vi "Boolean_Create.vi"(7 "Object Attributes":T1, 8 "error in (no error)":errorcluster, 9 "BooleanControl Attributes":T3, 10 "Control Attributes":T4, 11 "Boolean In":refnum<class "Boolean.lvclass">) -> (0 "error out":errorcluster, 3 "Boolean Out":refnum<class "Boolean.lvclass">)   [LabVIEW 2015, in "Front Panel Publisher.lvlib" / "Boolean.lvclass"]
uses:
  Boolean.lvclass
  Control_class/Attributes.ctl
  Text_class/Text.lvclass
  Attributes.ctl
  Object_class/Attributes.ctl
  Object_class/Coordinates.ctl
  Control_class/Control.lvclass
  Object_class/Object.lvclass
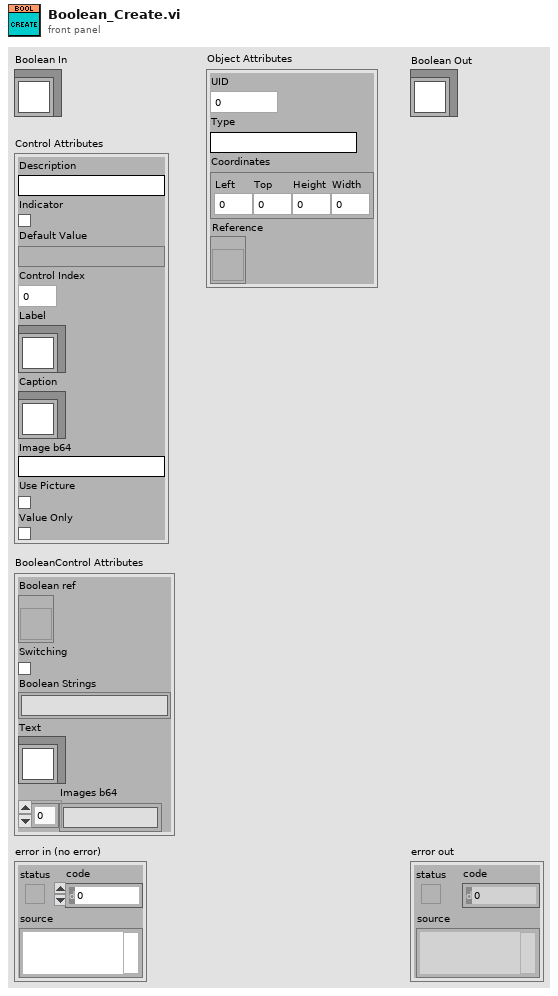
[diagram p1: front panel]
types:
  T1 = typedef "Front Panel Publisher.lvlib/Object.lvclass/Attributes.ctl" = cluster{"UID":i32, "Type":string, "Coordinates":T2, "Reference":refnum<vi>}
  T2 = typedef "Front Panel Publisher.lvlib/Object.lvclass/Coordinates.ctl" = cluster{"Left":i32, "Top":i32, "Height":u32, "Width":u32}
  T3 = typedef "Front Panel Publisher.lvlib/Boolean.lvclass/Attributes.ctl" = cluster{"Boolean ref":refnum<vi>, "Switching":bool, "Boolean Strings":string[], "Text":refnum<class "Text.lvclass">, "Images b64":string[]}
  T4 = typedef "Front Panel Publisher.lvlib/Control.lvclass/Attributes.ctl" = cluster{"Description":string, "Indicator":bool, "Default Value":variant, "Control Index":i32, "Label":refnum<class "Text.lvclass">, "Caption":refnum<class "Text.lvclass">, "Image b64":string, "Use Picture":bool, "Value Only":bool}
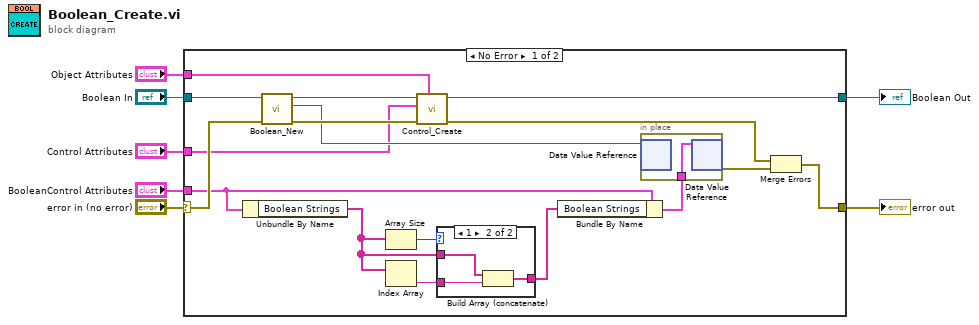
[diagram p0: block diagram]
diagram:
  n1 = case shown="No Error" "error in (no error)" {
    selector: "error in (no error)" -> [w24 w31]
    tunnel: [w22 w31] -> w6
    tunnel: "Boolean In" -> [w15 w30]
    tunnel: [w19 w30] -> w4
    tunnel: "Control Attributes" -> [w17 _]
    tunnel: "BooleanControl Attributes" -> [w10 _]
    tunnel: "Object Attributes" -> [w14 _]
    frame No Error {
      n2 = Unbundle By Name(w10) -> ("Boolean Strings"=w12:string[])
      n3 = call "Boolean_New.vi"("error in (no error)"=w24, "reference in"=w15) -> ("error out"=w20:errorcluster, "DVRRefOut"=w18:refnum<data-value>, "reference out"=w21:refnum<class "Boolean.lvclass">)  [unwired: 6 in, 1 out]
      n4 = Array Size(array=w12) -> (size(s)=w13:i32)
      n5 = Index Array(array=w12) -> (element=w11:string)  [unwired: 1 in]
      n6 = call "Control_Create.vi"("Object Attributes"=w14, "error in (no error)"=w20, "Control Attributes"=w17, "Control In"=w21) -> ("error out"=w16:errorcluster, "Control Out"=w19:refnum<class "Boolean.lvclass">)  [unwired: 6 in]
      n7 = case shown="1" w13 {
        tunnel: w12 -> [w25 w28]
        tunnel: w11 -> [_ w27]
        tunnel: [w25 w26] -> w8
        frame Default {
        }
        frame 1 {
          n8 = Build Array (concatenate)(w28, w27) -> (w26:string[])
        }
      }
      n9 = Bundle By Name(cluster=w10, "Boolean Strings"=w8) -> (w9:T3)
      n10 = in-place {
        in-place-border: w9 -> [w29]
        n11 = in-place-dvr #1(w18) -> ()  [unwired: 2 out]
        n12 = in-place-dvr #1(w29) -> (w23:errorcluster)  [unwired: 1 out]
      }
      n13 = Merge Errors(w16, w23) -> (w22:errorcluster)
    }
    frame Error {
    }
  }
  "error out" <- w6
  "Boolean Out" <- w4
